vi "moving average.vi"(1 "length":i32=10, 2 "raw array":dbl[](array[numeric])) -> (0 "averaged array":dbl[](array[numeric]))   [LabVIEW 2018, in "Sandbox.lvlib"]
uses:
  <vilib>/Analysis/baseanly.llb/Mean (DBL).vi
  Sandbox.lvlib
  <vilib>/Analysis/NI_AALBase.lvlib
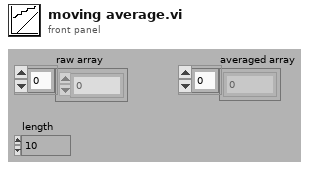
[diagram p1: front panel]
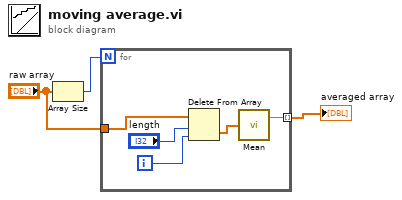
[diagram p0: block diagram]
diagram:
  n1 = Array Size(array="raw array") -> (size(s)=w1:i32)
  n2 = for {
    N: w1 -> [_]
    tunnel: "raw array" -> [w7]
    tunnel: [w5] -> w3 mode=indexing
    i -> [w8]
    n3 = Delete From Array "Delete From Array"(array=w7, length="length", index=w8) -> (deleted portion=w4:dbl[])  [unwired: 1 out]
    n4 = call-poly <vilib>:"Mean.vi"("X"=w4) -> ("mean"=w5:dbl)  [unwired: 1 out]
  }
  "averaged array" <- w3
